vi "Create Sysdef Tree from DB Channel Clusters.vi"(7 "Autocreate Rx timestamp chans?":bool, 8 "error in":errorcluster, 10 "channels":T1[](array[typedef]), 11 "Device Ptr":u64) -> (0 "error out":errorcluster, 3 "Device Ptr dup":u64)   [LabVIEW 2017, in "Ballard 1553 System Explorer.lvlib"]
uses:
  Ballard 1553 System Explorer.lvlib
  Parse XML Ballard/Ballard_Channel.ctl
  Parse XML Ballard/Ballard_BC.ctl
  Parse XML Ballard/Ballard_message.ctl
  Parse XML Ballard/Ballard_messageType.ctl
  Parse XML Ballard/Ballard_CWD1.ctl
  Parse XML Ballard/Ballard_CWD2.ctl
  Parse XML Ballard/Ballard_minorFrame.ctl
  Parse XML Ballard/Ballard_majorFrame.ctl
  Parse XML Ballard/Ballard_acyclicFrame.ctl
  Parse XML Ballard/Ballard_RT.ctl
  Parse XML Ballard/Ballard_RT subAddress.ctl
  Parse XML Ballard/Ballard_RT direction.ctl
  Parse XML Ballard/Ballard_RT rtMode.ctl
  Parse XML Ballard/Ballard_RT modeCode.ctl
  Shared/Controls and Global/Global.vi
  <vilib>/NI VeriStand/Custom Device API/Custom Device API.lvlib
  Shared/Ballard 1553 Shared.lvlib
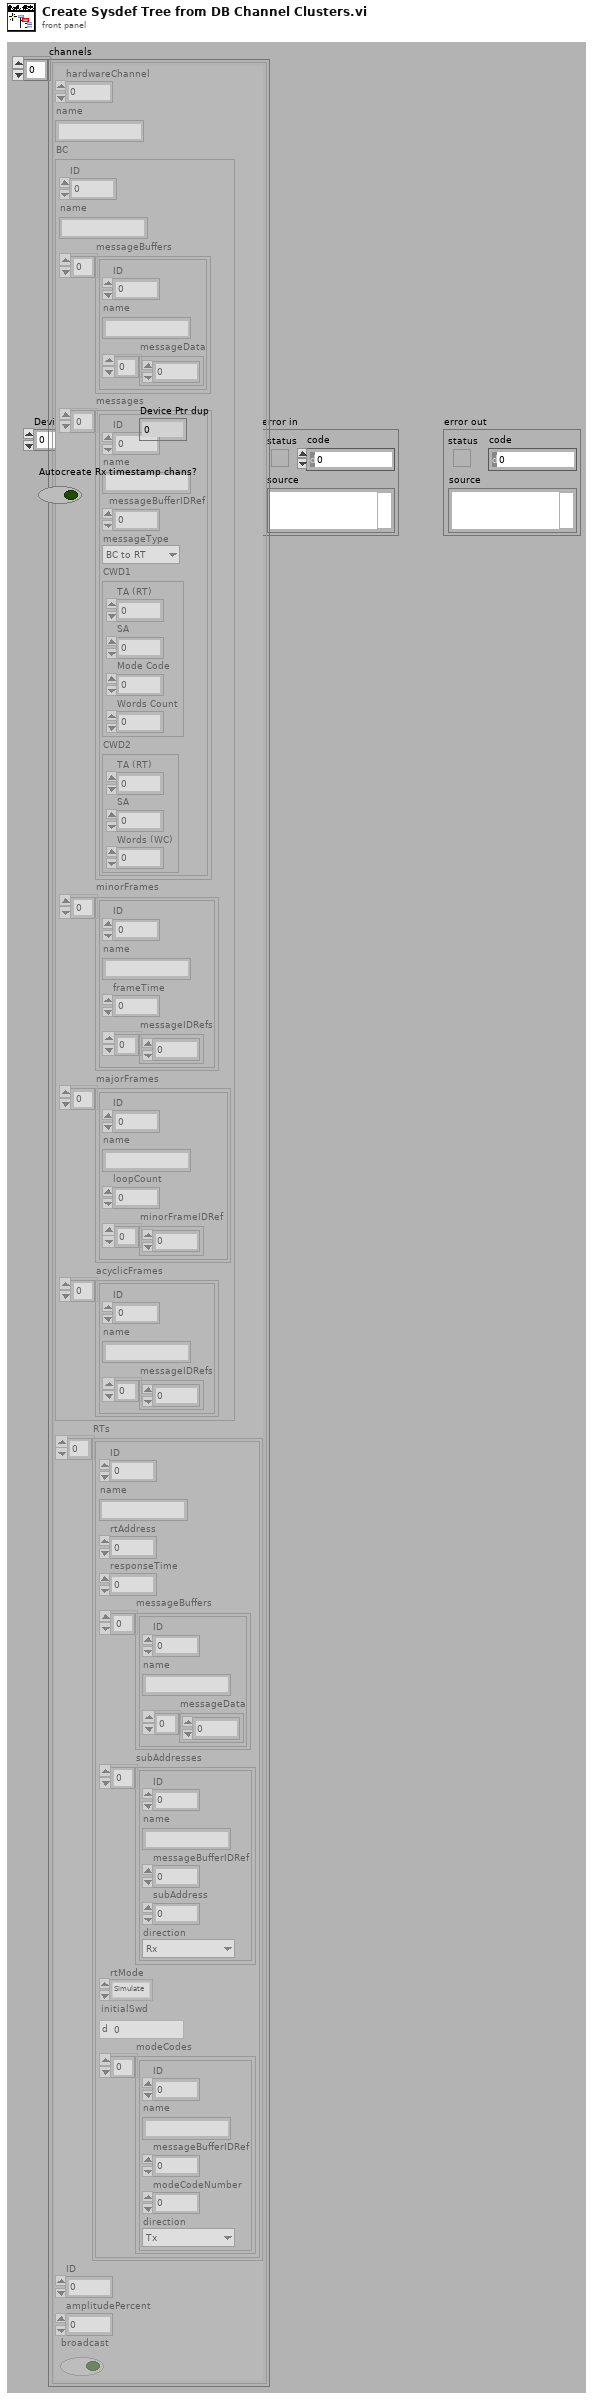
[diagram p1: front panel]
types:
  T1 = typedef "Ballard 1553 System Explorer.lvlib/Ballard_Channel.ctl" = cluster{"hardwareChannel":i32, "name":string, "BC":T2, "RTs":T10[], "ID":i32, "amplitudePercent":dbl, "broadcast":bool}
  T2 = typedef "Ballard 1553 System Explorer.lvlib/Ballard_BC.ctl" = cluster{"ID":i32, "name":string, "messageBuffers":cluster{"ID":i32, "name":string, "messageData":u16[]}[], "messages":T3[], "minorFrames":T7[], "majorFrames":T8[], "acyclicFrames":T9[]}
  T3 = typedef "Ballard 1553 System Explorer.lvlib/Ballard_message.ctl" = cluster{"ID":i32, "name":string, "messageBufferIDRef":i32, "messageType":T4, "CWD1":T5, "CWD2":T6}
  T4 = typedef "Ballard 1553 System Explorer.lvlib/Ballard_messageType.ctl" = enum16{"BC to RT", "RT to BC", "RT to RT", "MC (Rx)", "MC (Tx)"}
  T5 = typedef "Ballard 1553 System Explorer.lvlib/Ballard_CWD1.ctl" = cluster{"TA (RT)":i8, "SA":i8, "Mode Code":i8, "Words Count":i8}
  T6 = typedef "Ballard 1553 System Explorer.lvlib/Ballard_CWD2.ctl" = cluster{"TA (RT)":i8, "SA":i8, "Words (WC)":i8}
  T7 = typedef "Ballard 1553 System Explorer.lvlib/Ballard_minorFrame.ctl" = cluster{"ID":i32, "name":string, "frameTime":i32, "messageIDRefs":i32[]}
  T8 = typedef "Ballard 1553 System Explorer.lvlib/Ballard_majorFrame.ctl" = cluster{"ID":i32, "name":string, "loopCount":i32, "minorFrameIDRef":i32[]}
  T9 = typedef "Ballard 1553 System Explorer.lvlib/Ballard_acyclicFrame.ctl" = cluster{"ID":i32, "name":string, "messageIDRefs":i32[]}
  T10 = typedef "Ballard 1553 System Explorer.lvlib/Ballard_RT.ctl" = cluster{"ID":i32, "name":string, "rtAddress":i8, "responseTime":i32, "messageBuffers":cluster{"ID":i32, "name":string, "messageData":u16[]}[], "subAddresses":T11[], "rtMode":T13, "initialSwd":u16, "modeCodes":T14[]}
  T11 = typedef "Ballard 1553 System Explorer.lvlib/Ballard_RT subAddress.ctl" = cluster{"ID":i32, "name":string, "messageBufferIDRef":i32, "subAddress":i8, "direction":T12}
  T12 = typedef "Ballard 1553 System Explorer.lvlib/Ballard_RT direction.ctl" = enum16{"Tx", "Rx"}
  T13 = typedef "Ballard 1553 System Explorer.lvlib/Ballard_RT rtMode.ctl" = enum16{"Simulate", "Monitor", "Disable"}
  T14 = typedef "Ballard 1553 System Explorer.lvlib/Ballard_RT modeCode.ctl" = cluster{"ID":i32, "name":string, "messageBufferIDRef":i32, "modeCodeNumber":i8, "direction":T12}
  T15 = typedef "Custom Device API.lvlib/Custom Device Item Ref.ctl" = u64
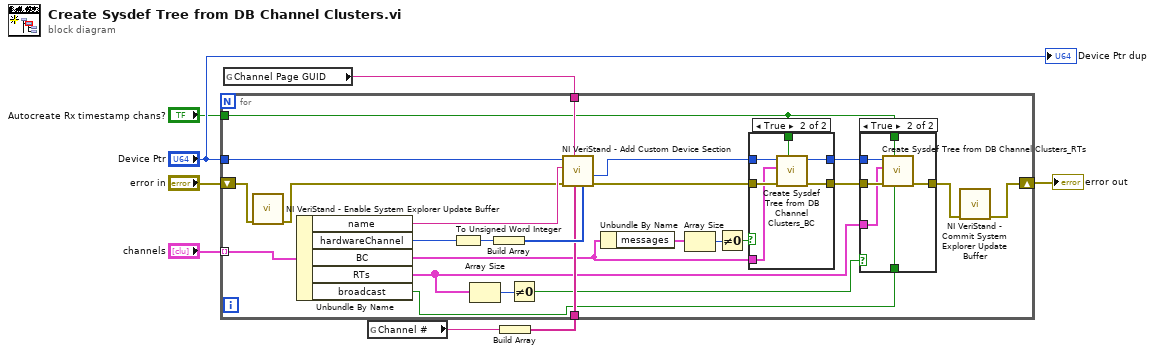
[diagram p0: block diagram]
diagram:
  n1 = global read "Global.vi" "Channel Page GUID"() -> (w2:string)
  n2 = global read "Global.vi" "Channel #"() -> (w1:string)
  n3 = Build Array(w1) -> (w7:string[])
  n4 = for {
    tunnel: "Device Ptr" -> [w31]
    shift-right: [w24] -> w5
    shift-left: "error in" -> [w26]
    tunnel: "channels" -> [w32] mode=indexing
    tunnel: w7 -> [w28]
    tunnel: "Autocreate Rx timestamp chans?" -> [w12]
    tunnel: w2 -> [w23]
    n5 = call <vilib>:"NI VeriStand - Enable System Explorer Update Buffer.vi"("error in (no error)"=w26) -> ("error out"=w25:errorcluster)  [unwired: 10 in]
    n6 = Unbundle By Name(w32) -> ("name"=w30:string, "hardwareChannel"=w29:i32, "BC"=w22:T2, "RTs"=w16:T10[], "broadcast"=w9:bool)
    n7 = To Unsigned Word Integer(number=w29) -> (unsigned 16bit integer=w27:u16)
    n8 = Array Size(array=w16) -> (size(s)=w20:i32)
    n9 = Build Array(w27) -> (w33:u16[])
    n10 = Not Equal To 0?(x=w20) -> (x != 0?=w17:bool)
    n11 = call <vilib>:"NI VeriStand - Add Custom Device Section.vi"("Property Values"=w33, "Property names"=w28, "GUID (Default Section)"=w23, "error in (no error)"=w25, "Section Name"=w30, "Parent Ref in"=w31) -> ("error out"=w21:errorcluster, "Section Ptr"=w13:T15)  [unwired: 2 in, 2 out]
    n12 = Unbundle By Name(w22) -> ("messages"=w10:T3[])
    n13 = Array Size(array=w10) -> (size(s)=w11:i32)
    n14 = Not Equal To 0?(x=w11) -> (x != 0?=w15:bool)
    n15 = case shown="True" w15 {
      tunnel: w22 -> [_ w44]
      tunnel: w21 -> [w42 w48]
      tunnel: [w42 w47] -> w19
      tunnel: w13 -> [w41 w46]
      tunnel: [w41 w45] -> w14
      tunnel: w12 -> [_ w43]
      frame False {
      }
      frame True {
        n16 = call "Create Sysdef Tree from DB Channel Clusters_BC.vi"("Autocreate Rx timestamp chans?"=w43, "error in"=w48, "BC"=w44, "Device Ptr"=w46) -> ("error out"=w47:errorcluster, "Device Ptr dup"=w45:u64)  [unwired: 6 in]
      }
    }
    n17 = case shown="True" w17 {
      tunnel: w19 -> [w34 w39]
      tunnel: [w34 w38] -> w18
      tunnel: w16 -> [_ w36]
      tunnel: w14 -> [_ w40]
      tunnel: w12 -> [_ w37]
      tunnel: w9 -> [_ w35]
      frame False {
      }
      frame True {
        n18 = call "Create Sysdef Tree from DB Channel Clusters_RTs.vi"("broadcast"=w35, "Autocreate Rx timestamp chans?"=w37, "error in"=w39, "RTs"=w36, "Device Ptr"=w40) -> ("error out"=w38:errorcluster)  [unwired: 6 in]
      }
    }
    n19 = call <vilib>:"NI VeriStand - Commit System Explorer Update Buffer.vi"("error in (no error)"=w18) -> ("error out"=w24:errorcluster)  [unwired: 10 in]
  }
  "error out" <- w5
  "Device Ptr dup" <- "Device Ptr"
